vi "Write.vi"(8 "error in (no error)":errorcluster, 10 "String":string, 11 "CLI Output in":refnum<class "CLI Output.lvclass">) -> (0 "error out":errorcluster, 3 "CLI Output out":refnum<class "CLI Output.lvclass">)   [LabVIEW 2019, in "CLI Output.lvclass"]
uses:
  CLI Output.lvclass
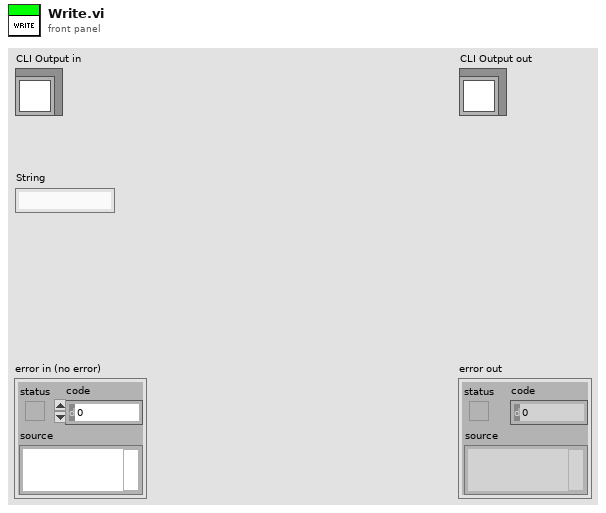
[diagram p1: front panel]
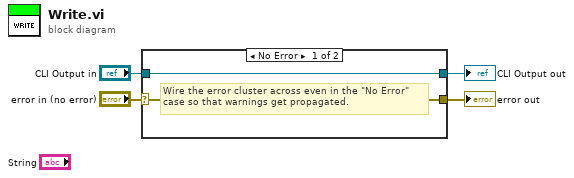
[diagram p0: block diagram]
diagram:
  n1 = case shown="No Error" "error in (no error)" {
    selector: "error in (no error)" -> [w5 w8]
    tunnel: [w5 w8] -> w3
    tunnel: [w6 w7] -> w1
    tunnel: "CLI Output in" -> [w6 w7]
    frame No Error {
      # "Wire the error cluster across even in the \"No Error\"\ncase so that warnings get propagated."
    }
    frame Error {
    }
  }
  "error out" <- w3
  "CLI Output out" <- w1
